vi "Onboard Archive.vi"() -> ()   [LabVIEW 2023]
doc: "This VI reads the \"Telemetry Recorder\" queue and writes it to either the SD card or USB flashdrive."
uses:
  <vilib>/Platform/TimedLoop/XDataNode/timing_clust.ctl
  <vilib>/Platform/TimedLoop/XDataNode/nitl_modes.ctl
  <vilib>/Platform/TimedLoop/XDataNode/wakeup.ctl
  Type Definitions/Payload Class.ctl
  Type Definitions/Enumerated Constants/Software Monitor.ctl
  Type Definitions/Data Frame.ctl
  Type Definitions/Data Frame Header.ctl
  Type Definitions/Device.ctl
  <vilib>/Utility/miscctls.llb/LVDateTimeRec.ctl
  Type Definitions/Enum - Notification Types.ctl
  <userlib>/_OpenG.lib/array/array.llb/Sort 1D Array (DBL)__ogtk.vi
  <userlib>/_OpenG.lib/array/array.llb/Reorder 1D Array2 (Path)__ogtk.vi
  <vilib>/platform/TimedLoop/XDataNode/XDataNode.xnode
  <vilib>/Platform/TimedLoop/XDataNode/XDNodeRunTimeDep.lvlib
  <userlib>/_OpenG.lib/array/array.llb/openg_array.lvlib
panel:
  out "All Files in Dir":path[](array[path])
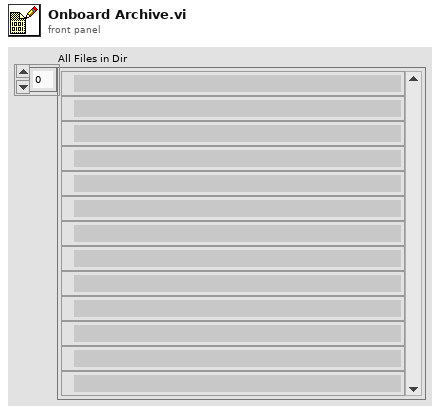
[diagram p1: front panel]
types:
  T1 = typedef "XDNodeRunTimeDep.lvlib/timing_clust.ctl" = cluster{"Expected End [f-1]":u64, "Actual End [f-1]":u64, "Finished Late? [f-1]":bool, "Expected End [i-1]":u64, "Actual End [i-1]":u64, "Finished Late? [i-1]":bool, "Expected Start [i]":u64, "Actual Start [i]":u64, "Expected Start [f]":u64, "Actual Start [f]":u64, "Source Name":string, "Structure Name":string, "Period":i64, "Deadline":i64, "Offset":i64, "Start":i64, "Priority":i32, "Timeout":i32, "Mode":T2, "Wakeup Reason":T3, "Error":errorcluster, "Source Type":string, "Secondary Source Type":string, "Global End Time":u64, "Global Start Time":u64, "Frame Duration":u64, "Iteration Duration":u64, "Assigned CPU":i32, "I/O Scan Engine Mode":u32}
  T2 = typedef "XDNodeRunTimeDep.lvlib/nitl_modes.ctl" = enum32{"No Change", "Process missed periods, maintain original phase", "Discard missed periods, maintain original phase", "Process missed periods, ignore original phase", "Discard missed periods, ignore original phase"}
  T3 = typedef "XDNodeRunTimeDep.lvlib/wakeup.ctl" = enum32{"Normal", "Aborted", "Asynchronous wakeup", "Timing source error", "Timed loop error", "Timeout"}
  T4 = typedef "Enum - Notification Types.ctl" = enum16{"Warning", "Acknowledge", "Notification"}
  T5 = typedef "LVDateTimeRec.ctl" = cluster{"fractional second":dbl, "second":i32, "minute":i32, "hour":i32, "day of month":i32, "month":i32, "year":i32, "day of week":i32, "day of year":i32, "DST":i32}
  T6 = typedef "Disk State.ctl" = cluster{"File System Name":string, "Total":sgl, "Available":sgl, "Used":sgl, "Path":string}
  T7 = typedef "Software Monitor.ctl" = enum16{"Internet Connection Monitor", "CPU Monitor", "Archive Monitor", "Memory Monitor", "Queue Monitor", "RTOS Update", "RTOS Monitor"}
  T8 = typedef "Payload Class.ctl" = enum16{"System State", "Parameters", "Metadata", "Software Monitor", "Data", "Commands"}
  T9 = typedef "Data Frame.ctl" = cluster{"Frame Header":T10, "Payload":string, "CRC":u32}
  T10 = typedef "Data Frame Header.ctl" = cluster{"Sync":u32, "Time":dbl, "Nanosecond Counter":i64, "Payload Class":T8, "Payload ID":u16, "Counter":i32, "Options":u32, "Source":T11, "Destination":T11}
  T11 = typedef "Device.ctl" = enum32{"None", "Exec", "Aux1", "Aux2", "Aux3"}
  T12 = typedef "Telemetry Recorder Status.ctl" = cluster{"Filepath":string, "File Size":i64, "Frame Count":i32, "Mean MB/hour":sgl}
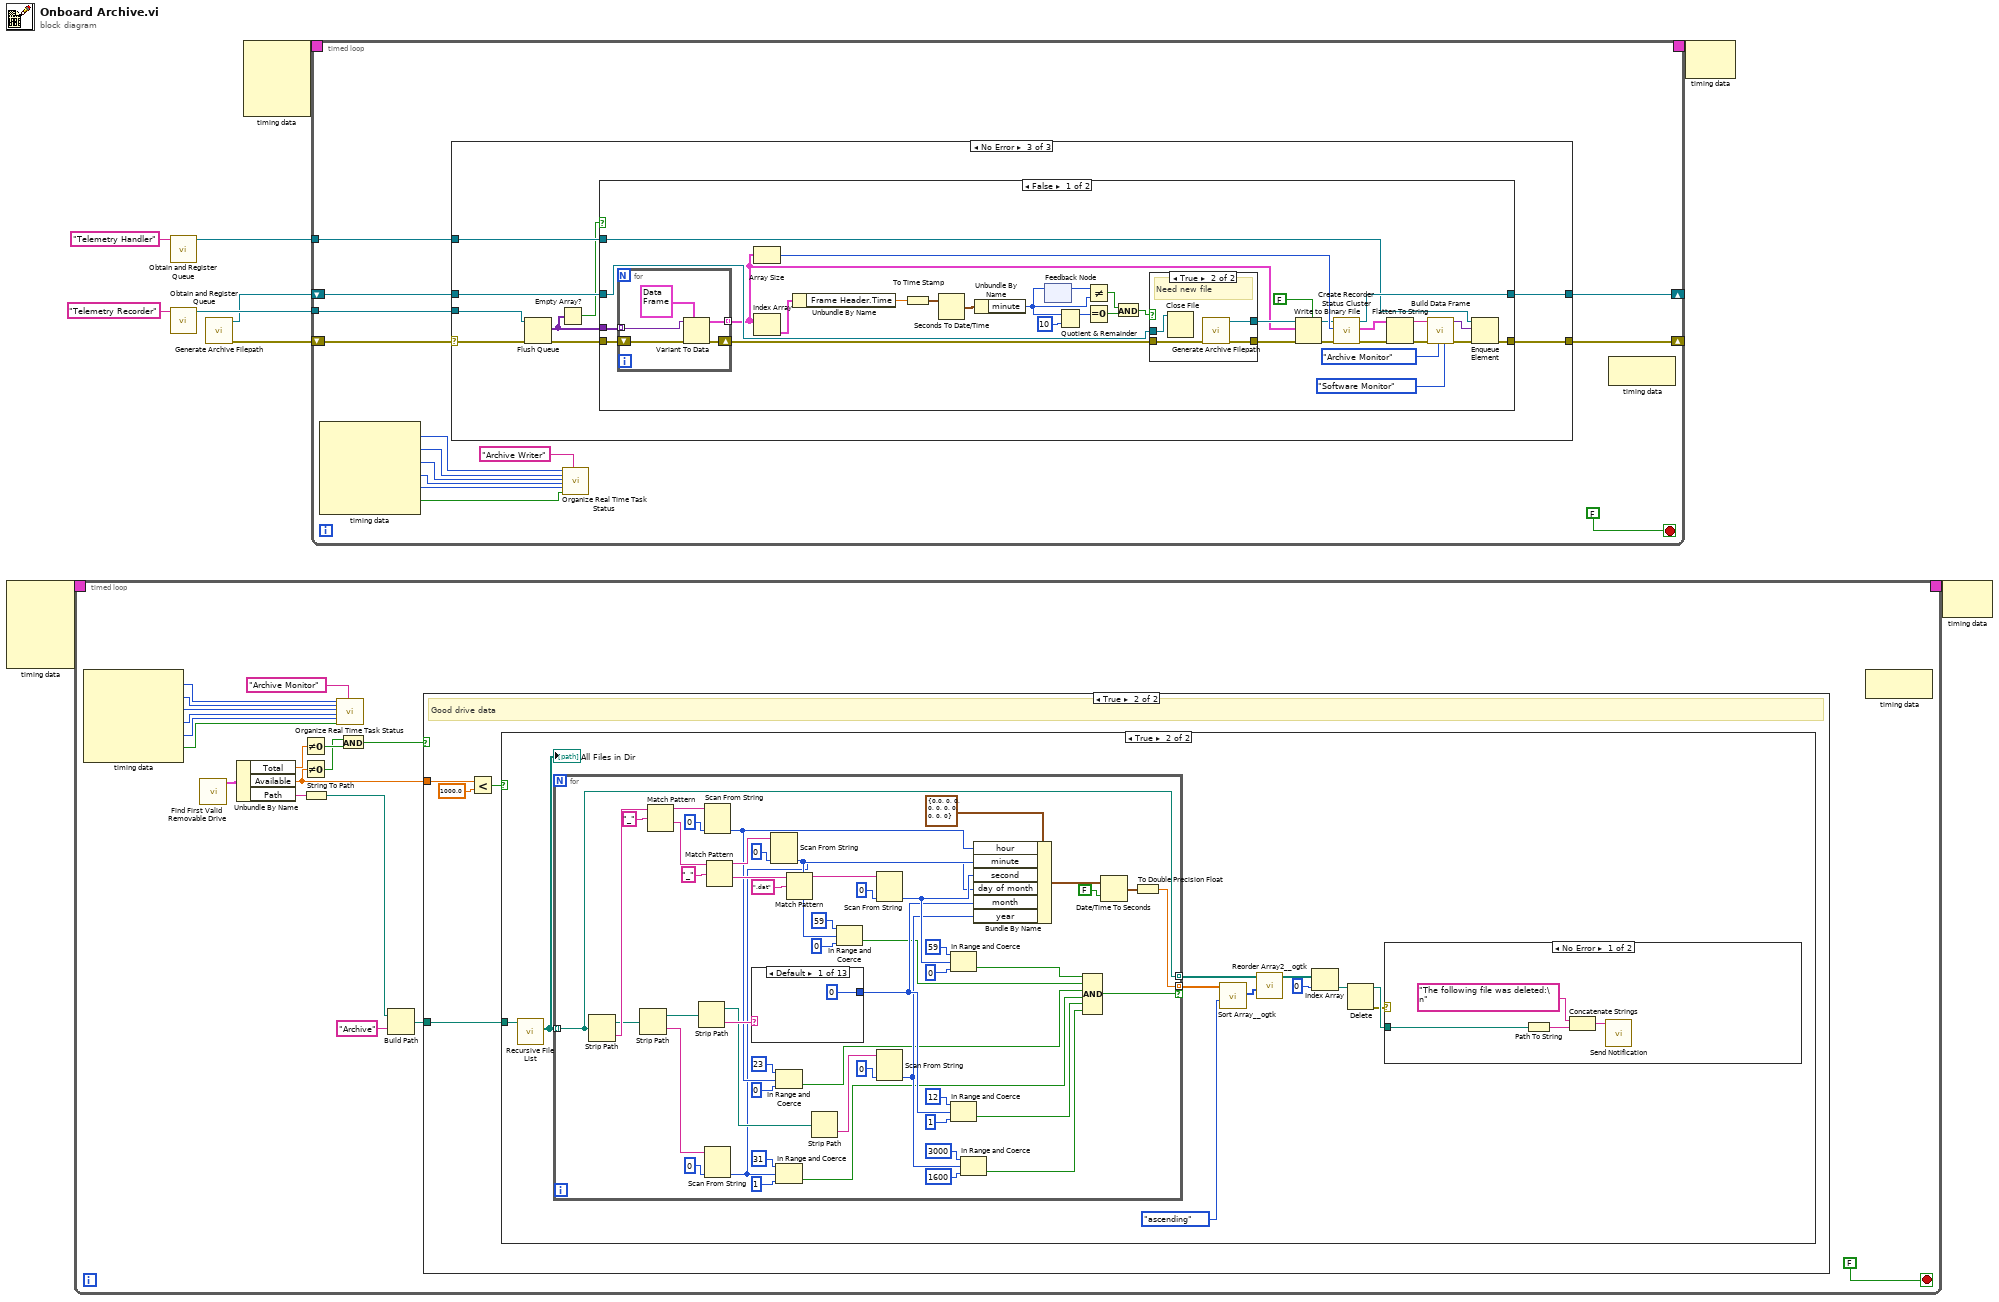
[diagram p0: block diagram]
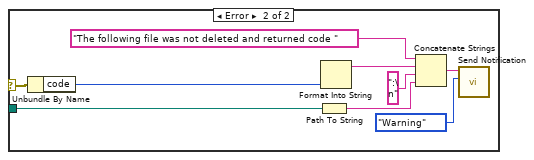
[diagram p4: hidden frame]
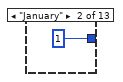
[diagram p5: hidden frame]
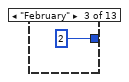
[diagram p6: hidden frame]
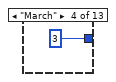
[diagram p7: hidden frame]
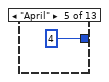
[diagram p8: hidden frame]
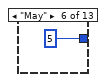
[diagram p9: hidden frame]
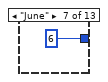
[diagram p10: hidden frame]
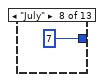
[diagram p11: hidden frame]
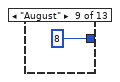
[diagram p12: hidden frame]
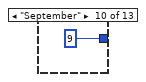
[diagram p13: hidden frame]
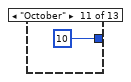
[diagram p14: hidden frame]
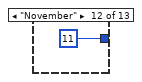
[diagram p15: hidden frame]
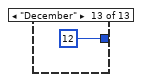
[diagram p16: hidden frame]
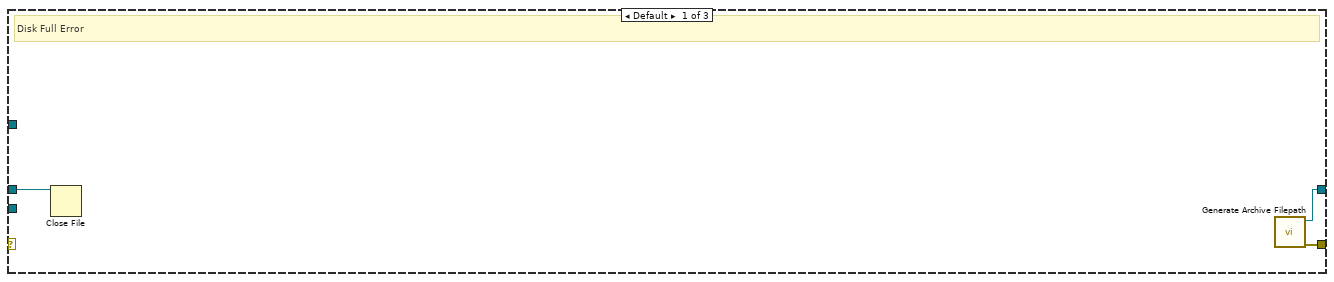
[diagram p17: hidden frame]
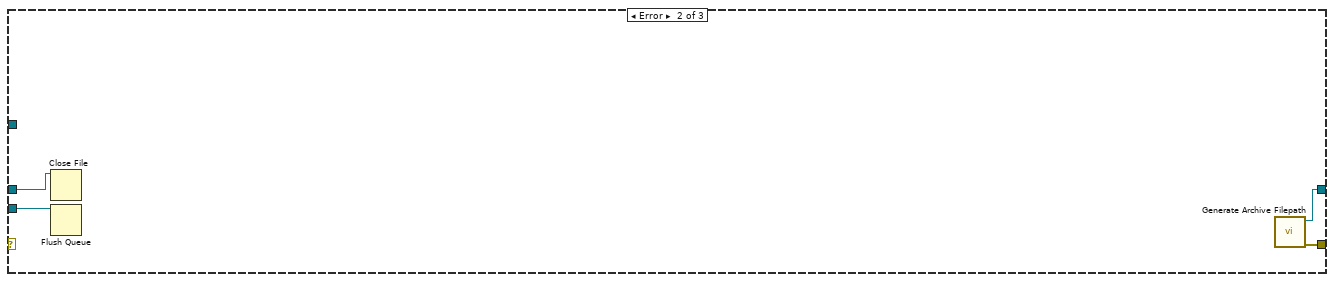
[diagram p18: hidden frame]
diagram:
  n1 = node-c288() -> (w2:T1)  [unwired: 5 in]
  n2 = timed-loop {
    timing: w2 -> [_]
    timing-out: [_] -> w1
    stop <- FALSE stop-if-true
    n3 = node-c288() -> (w16:i32, w15:i32, w14:i64, w13:i64, w12:i64, w11:bool)  [unwired: 1 in]
    n4 = call "Find First Valid Removable Drive.vi"() -> ("Disk State"=w24:T6)  [unwired: 11 in]
    n5 = Unbundle By Name(w24) -> ("Total"=w23:sgl, "Available"=w18:sgl, "Path"=w22:string)
    n6 = Not Equal To 0?(x=w23) -> (x != 0?=w27:bool)
    n7 = Not Equal To 0?(x=w18) -> (x != 0?=w26:bool)
    n8 = String To Path(string=w22) -> (path=w20:path)
    n9 = call "Organize Real Time Task Status.vi"("Priority"=w16, "Processor"=w15, "Offset"=w14, "Iteration Duration"=w13, "Period"=w12, "Finished Late? [i-1]"=w11, "Task Name"="Archive Monitor") -> ()  [unwired: 12 in, 1 out]
    n10 = And(x=w26, y=w27) -> (x .and. y?=w25:bool)
    n11 = Build Path(base path=w20, name or relative path="Archive" ("Path")) -> (appended path=w19:path)
    n12 = case shown="True" w25 {
      tunnel: w18 -> [_ w32]
      tunnel: w19 -> [_ w29]
      frame False {
        # "Bad drive data"
      }
      frame True {
        # "Good drive data"
        n13 = Less?(x=w32, y=sgl 1000.0) -> (x < y?=w30:bool)
        n14 = case shown="True" w30 {
          tunnel: w29 -> [_ w34]
          frame False {
          }
          frame True {
            n15 = call <vilib>:"Recursive File List.vi"("Folder Path"=w34) -> ("All Files in Dir"=w43:path[])  [unwired: 6 in, 4 out]
            "All Files in Dir" <- w43
            n16 = for {
              tunnel: w43 -> [w82] mode=indexing
              tunnel: [w83] -> w41 mode=indexing if=w57
              tunnel: [w82] -> w40 mode=indexing
              n17 = Strip Path(path=w82) -> (stripped path=w94:path, name=w107:string)
              n18 = Strip Path(path=w94) -> (stripped path=w91:path, name=w92:string)
              n19 = Match Pattern(string=w107, regular expression="_") -> (before substring=w95:string, after substring=w105:string)  [unwired: 1 in, 2 out]
              n20 = Strip Path(path=w91) -> (stripped path=w89:path, name=w90:string)
              n21 = Scan From String(input string=w95, default 1=0 ("hour")) -> (output 1=w73:i32)  [unwired: 3 in, 3 out]
              n22 = Scan From String(input string=w92, default 1=0 ("hour")) -> (output 1=w70:i32)  [unwired: 3 in, 3 out]
              n23 = Match Pattern(string=w105, regular expression="_") -> (before substring=w97:string, after substring=w103:string)  [unwired: 1 in, 2 out]
              n24 = case shown="Default" w90 {
                tunnel: [0 ("hour") 1 ("hour") 2 ("hour") 3 ("hour") 4 ("hour") 5 ("hour") 6 ("hour") 7 ("hour") 8 ("hour") 9 ("hour") 10 ("hour") 11 ("hour") 12 ("hour")] -> w67
                frame Default {
                }
                frame "January" {
                }
                frame "February" {
                }
                frame "March" {
                }
                frame "April" {
                }
                frame "May" {
                }
                frame "June" {
                }
                frame "July" {
                }
                frame "August" {
                }
                frame "September" {
                }
                frame "October" {
                }
                frame "November" {
                }
                frame "December" {
                }
              }
              n25 = Scan From String(input string=w97, default 1=0 ("hour")) -> (output 1=w76:i32)  [unwired: 3 in, 3 out]
              n26 = In Range and Coerce(upper limit=23, x=w73, lower limit=0) -> (In Range?=w61:bool)  [unwired: 1 out]
              n27 = In Range and Coerce(upper limit=31, x=w70, lower limit=1) -> (In Range?=w60:bool)  [unwired: 1 out]
              n28 = Match Pattern(string=w103, regular expression=".dat") -> (before substring=w96:string)  [unwired: 1 in, 3 out]
              n29 = Strip Path(path=w89) -> (name=w87:string)  [unwired: 1 out]
              n30 = In Range and Coerce(upper limit=59, x=w76, lower limit=0) -> (In Range?=w62:bool)  [unwired: 1 out]
              n31 = Scan From String(input string=w96, default 1=0 ("hour")) -> (output 1=w81:i32)  [unwired: 3 in, 3 out]
              n32 = Scan From String(input string=w87, default 1=0 ("hour")) -> (output 1=w64:i32)  [unwired: 3 in, 3 out]
              n33 = In Range and Coerce(upper limit=59, x=w81, lower limit=0) -> (In Range?=w63:bool)  [unwired: 1 out]
              n34 = In Range and Coerce(upper limit=12, x=w67, lower limit=1) -> (In Range?=w59:bool)  [unwired: 1 out]
              n35 = In Range and Coerce(upper limit=3000, x=w64, lower limit=1600) -> (In Range?=w58:bool)  [unwired: 1 out]
              n36 = Bundle By Name(cluster=T5 {"fractional second"=0.0, "second"=0, "minute"=0, "hour"=0, "day of month"=0, "month"=0, "year"=0, "day of week"=0, "day of year"=0, "DST"=0} ("date time rec"), "hour"=w73, "minute"=w76, "second"=w81, "day of month"=w70, "month"=w67, "year"=w64) -> (w86:T5)
              n37 = Compound Arithmetic op=AND(w63, w62, w61, w60, w59, w58) -> (w57:bool)
              n38 = Date/Time To Seconds(1:FALSE ("is UTC (F)"), 2:w86) -> (0:w84:timestamp)
              n39 = To Double Precision Float(number=w84) -> (double precision float=w83:dbl)
            }
            n40 = call-poly <userlib>:"Sort Array__ogtk.vi"("Order"=enum16{"ascending", "descending"}."ascending", "Array in"=w41) -> ("Sorted Pointers"=w39:i32[])  [unwired: 8 in, 1 out]
            n41 = call-poly <userlib>:"Reorder Array2__ogtk.vi"("indices"=w39, "array"=w40) -> ("reordered array"=w38:path[])  [unwired: 9 in]
            n42 = Index Array(array=w38, index=0) -> (element=w36:path)
            n43 = Delete(path (use dialog)=w36) -> (deleted path=w35:path, error out=w33:errorcluster)  [unwired: 4 in, 1 out]
            n44 = case shown="No Error" w33 {
              selector: w33 -> [_ w54]
              tunnel: w35 -> [w46 w56]
              frame No Error {
                n45 = Path To String(path=w46) -> (string=w45:string)
                n46 = Concatenate Strings("The following file was deleted:\n" ("Additional Message Details"), w45) -> (w44:string)
                n47 = call "Send Notification.vi"("Description (\"\")"=w44) -> ()  [unwired: 9 in, 2 out]
              }
              frame Error {
                n48 = Unbundle By Name(w54) -> ("code"=w53:i32)
                n49 = Path To String(path=w56) -> (string=w51:string)
                n50 = Format Into String(w53) -> (resulting string=w52:string)  [unwired: 3 in, 1 out]
                n51 = Concatenate Strings("The following file was not deleted and returned code " ("string"), w52, ":\n" ("string"), w51) -> (w49:string)
                n52 = call "Send Notification.vi"("Notification Type (Notification)"=Enum_-_Notification_Types."Warning", "Description (\"\")"=w49) -> ()  [unwired: 8 in, 2 out]
              }
            }
          }
        }
      }
    }
    n53 = node-c288() -> ()  [unwired: 1 in, 1 out]
  }
  n54 = call "Obtain and Register Queue.vi"("Queue Name (unnamed)"="Telemetry Handler" ("name (unnamed)")) -> ("Queue Reference"=w8:refnum<queue>)  [unwired: 9 in, 1 out]
  n55 = call "Obtain and Register Queue.vi"("Queue Name (unnamed)"="Telemetry Recorder" ("name (unnamed)")) -> ("Queue Reference"=w6:refnum<queue>)  [unwired: 9 in, 1 out]
  n56 = call "Generate Archive Filepath.vi"() -> ("error out"=w3:errorcluster, "File Reference"=w4:refnum<file>)  [unwired: 9 in, 1 out]
  n57 = node-c288() -> (w10:T1)  [unwired: 4 in]
  n58 = timed-loop {
    tunnel: w6 -> [w142]
    shift-right: [w140] -> _
    shift-left: w3 -> [w137]
    shift-right: [w139] -> _
    shift-left: w4 -> [w138]
    timing: w10 -> [_]
    timing-out: [_] -> w9
    tunnel: w8 -> [w136]
    stop <- FALSE stop-if-true
    n59 = node-c288() -> (w134:i32, w133:i32, w132:i64, w131:i64, w130:i64, w129:bool)  [unwired: 1 in]
    n60 = case shown="No Error" w137 {
      selector: w137 -> [_ _ w164]
      tunnel: w142 -> [_ w156 w165]
      tunnel: [w151 w154 w161] -> w140
      tunnel: [w152 w155 w162] -> w139
      tunnel: w138 -> [w153 w157 w166]
      tunnel: w136 -> [_ _ w160]
      frame Default {
        # "Disk Full Error"
        n61 = Close File(refnum=w153) -> ()  [unwired: 1 in, 2 out]
        n62 = call "Generate Archive Filepath.vi"() -> ("error out"=w151:errorcluster, "File Reference"=w152:refnum<file>)  [unwired: 9 in, 1 out]
      }
      frame Error {
        n63 = Close File(refnum=w157) -> ()  [unwired: 1 in, 2 out]
        n64 = Flush Queue(queue=w156) -> ()  [unwired: 1 in, 3 out]
        n65 = call "Generate Archive Filepath.vi"() -> ("error out"=w154:errorcluster, "File Reference"=w155:refnum<file>)  [unwired: 9 in, 1 out]
      }
      frame No Error {
        n66 = Flush Queue(queue=w165, error in (no error)=w164) -> (remaining elements=w159:variant[], error out=w163:errorcluster)  [unwired: 1 out]
        n67 = Empty Array?(array=w159) -> (empty?=w158:bool)
        n68 = case shown="False" w158 {
          tunnel: w166 -> [w199 w211]
          tunnel: w163 -> [w197 w212]
          tunnel: w159 -> [w196 _]
          tunnel: [w184 w211] -> w162
          tunnel: [w176 w212] -> w161
          tunnel: w160 -> [w175 _]
          frame False {
            n69 = for {
              tunnel: [w209] -> w171 mode=indexing
              tunnel: w196 -> [w206] mode=indexing
              shift-right: [w208] -> w198
              shift-left: w197 -> [w207]
              n70 = Variant To Data(error in=w207, type=T9 {"Frame Header"={"Sync"=0, "Time"=0.0, "Nanosecond Counter"=0, "Payload Class"=enum."System State", "Payload ID"=0, "Counter"=0, "Options"=0, "Source"=enum."None", "Destination"=enum."None"}, "Payload"="", "CRC"=0} ("Frame"), Variant=w206) -> (data=w209:T9, error out=w208:errorcluster)
            }
            n71 = Array Size(array=w171) -> (size(s)=w183:i32)
            n72 = Index Array(array=w171) -> (element=w185:T9)  [unwired: 1 in]
            n73 = Unbundle By Name(w185) -> ("Frame Header.Time"=w188:dbl)
            n74 = To Time Stamp(1:w188) -> (0:w187:timestamp)
            n75 = Seconds To Date/Time(time stamp (now)=w187) -> (date time rec=w195:T5)  [unwired: 1 in]
            n76 = Unbundle By Name(w195) -> ("minute"=w193:i32)
            n77 = feedback #1() -> (w192:i32)  [unwired: 1 in]
            n78 = feedback-in #1(w193) -> ()
            n79 = Quotient & Remainder(x=w193, y=10) -> (x-y*floor(x/y)=w190:i32)  [unwired: 1 out]
            n80 = Not Equal?(x=w192, y=w193) -> (x != y?=w194:bool)
            n81 = Equal To 0?(x=w190) -> (x = 0?=w191:bool)
            n82 = And(x=w194, y=w191) -> (x .and. y?=w186:bool)
            n83 = case shown="True" w186 {
              tunnel: [w200 w203] -> w173
              tunnel: w198 -> [w200 w204]
              tunnel: [w201 w202] -> w172
              tunnel: w199 -> [w201 w205]
              frame False {
                # "Current File is Good"
              }
              frame True {
                # "Need new file"
                n84 = Close File(refnum=w205) -> ()  [unwired: 1 in, 2 out]
                n85 = call "Generate Archive Filepath.vi"("error in (no error)"=w204) -> ("error out"=w203:errorcluster, "File Reference"=w202:refnum<file>)  [unwired: 8 in, 1 out]
              }
            }
            n86 = Write to Binary File(file (use dialog)=w172, data=w171, error in=w173, 5:FALSE ("prepend array or string size? (T)")) -> (refnum out=w170:refnum<file>, error out=w169:errorcluster)  [unwired: 2 in, 1 out]
            n87 = call "Create Recorder Status Cluster.vi"("error in (no error)"=w169, "Frames Written this iteration"=w183, "File Reference In"=w170) -> ("error out"=w178:errorcluster, "Data Recorder Status"=w180:T12, "File Reference Out"=w184:refnum<file>)  [unwired: 6 in]
            n88 = Flatten To String(anything=w180, error in (no error)=w178) -> (data string=w182:string, error out=w181:errorcluster)  [unwired: 2 in, 1 out]
            n89 = call "Build Data Frame.vi"("Payload Class (Data)"=Payload_Class."Software Monitor", "Payload ID (0)"=Software_Monitor."Archive Monitor" ("Software Monitor"), "error in (no error)"=w181, "Payload (Empty String)"=w182) -> ("error out"=w177:errorcluster, "Frame"=w174:variant)  [unwired: 6 in]
            n90 = Enqueue Element(queue=w175, element=w174, error in (no error)=w177) -> (error out=w176:errorcluster)  [unwired: 1 in, 2 out]
          }
          frame True {
            # "Empty archive queue"
          }
        }
      }
    }
    n91 = call "Organize Real Time Task Status.vi"("Priority"=w134, "Processor"=w133, "Offset"=w132, "Iteration Duration"=w131, "Period"=w130, "Finished Late? [i-1]"=w129, "Task Name"="Archive Writer") -> ()  [unwired: 12 in, 1 out]
    n92 = node-c288() -> ()  [unwired: 1 in, 1 out]
  }
  n93 = node-c288(w9) -> ()  [unwired: 1 out]
  n94 = node-c288(w1) -> ()  [unwired: 1 out]
